vi "GetNodeID.vi"(11 "UDP_Config in":refnum<class "UDP_Config.lvclass">) -> (2 "NodeID":string, 3 "UDP_Config out":refnum<class "UDP_Config.lvclass">)   [LabVIEW 2021, in "UDP_Config.lvclass"]
uses:
  UDP_Config.lvclass
  UDP_Config.lvclass/UDP_Config.ctl
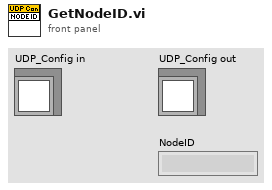
[diagram p1: front panel]
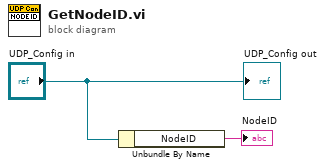
[diagram p0: block diagram]
diagram:
  n1 = Unbundle By Name("UDP_Config in") -> ("NodeID"=→"NodeID":string)
  "UDP_Config out" <- "UDP_Config in"
